vi "LoadServerCfg.vi"(8 "error in (no error)":errorcluster, 11 "RESTLoaderConstant in":refnum<class "RESTLoaderConstant.lvclass">) -> (0 "error out":errorcluster, 2 "Server config":T1={"API Root"="", "verify server"=FALSE, "Version (no version)"="", "Port (protocol specific)"=0, "Base URL"="", "Auth type"=enum."Token", "Auth string"="", "timeout (10000)"=10000, "Token preamble (Token)"="", "Token empty preamble (False)"=FALSE, "Token header key (Authorization)"=""}, 3 "RESTLoaderConstant out":refnum<class "RESTLoaderConstant.lvclass">)   [LabVIEW 2019, in "ByteREST.lvlib" / "RESTLoaderConstant.lvclass"]
uses:
  RESTLoaderConstant.lvclass
  LoaderBase/ServerParams.ctl
  ByteRESTClass/ByteRESTBase/Auth/Authentication_type.ctl
  RESTLoaderConstant.lvclass/RESTLoaderConstant.ctl
  LoaderBase/RESTLoaderBase.lvclass
  ByteRESTClass/ByteRESTBase/RESTBase.lvclass
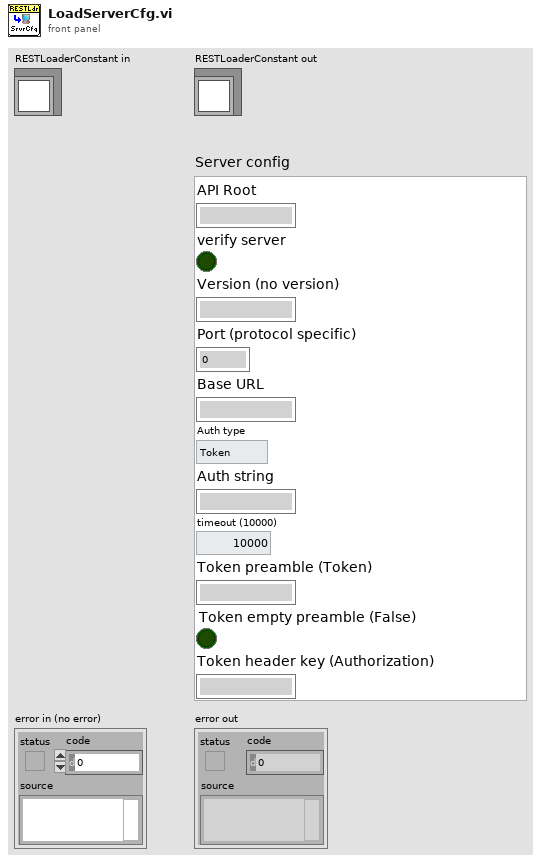
[diagram p1: front panel]
types:
  T1 = typedef "ByteREST.lvlib/RESTLoaderBase.lvclass/ServerParams.ctl" = cluster{"API Root":string, "verify server":bool, "Version (no version)":string, "Port (protocol specific)":u16, "Base URL":string, "Auth type":T2, "Auth string":string, "timeout (10000)":i32, "Token preamble (Token)":string, "Token empty preamble (False)":bool, "Token header key (Authorization)":string}
  T2 = typedef "ByteREST.lvlib/RESTBase.lvclass/Authentication_type.ctl" = enum16{"Token"}
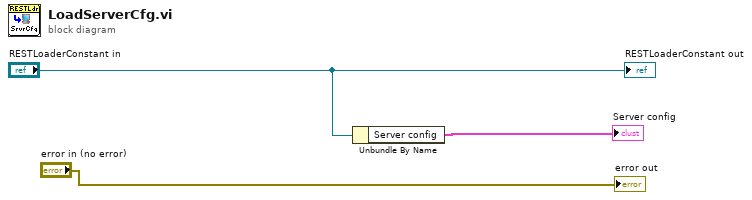
[diagram p0: block diagram]
diagram:
  n1 = Unbundle By Name("RESTLoaderConstant in") -> ("Server config"=→"Server config":T1)
  "error out" <- "error in (no error)"
  "RESTLoaderConstant out" <- "RESTLoaderConstant in"
